vi "pmu_Write Physical Channel Info.vi"(8 "error in (no error)":errorcluster, 10 "physical channels":T1[](array[typedef]), 11 "system info in":refnum<class "PMU System Info.lvclass">) -> (0 "error out":errorcluster, 3 "system info out":refnum<class "PMU System Info.lvclass">)   [LabVIEW 2011, in "NI_EP_PMU.lvlib" / "PMU System Info.lvclass"]
uses:
  <vilib>/addons/Electrical Power/PMU/Common/Classes/PMU System Info/PMU System Info.lvclass
  <vilib>/addons/Electrical Power/PMU/Common/Controls/pmu_Physical Channel.ctl
  <vilib>/addons/Electrical Power/PMU/Common/Controls/pmu_Channel Phase.ctl
  <vilib>/addons/Electrical Power/PMU/Common/Classes/PMU System Info/PMU System Info.lvclass/PMU System Info.ctl
  <vilib>/addons/Electrical Power/PMU/NI_EP_PMU.lvlib
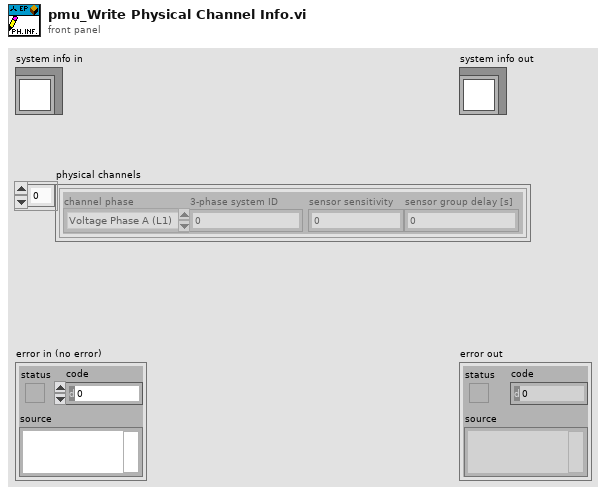
[diagram p1: front panel]
types:
  T1 = typedef "NI_EP_PMU.lvlib/pmu_Physical Channel.ctl" = cluster{"channel phase":T2, "3-phase system ID":u8, "sensor sensitivity":dbl, "sensor group delay [s]":dbl}
  T2 = typedef "NI_EP_PMU.lvlib/pmu_Channel Phase.ctl" = enum16{"Voltage Phase A (L1)", "Voltage Phase B (L2)", "Voltage Phase C (L3)", "Voltage Phase N (Neutral)", "Current Phase A (L1)", "Current Phase B (L2)", "Current Phase C (L3)", "Current Phase N (Neutral)"}
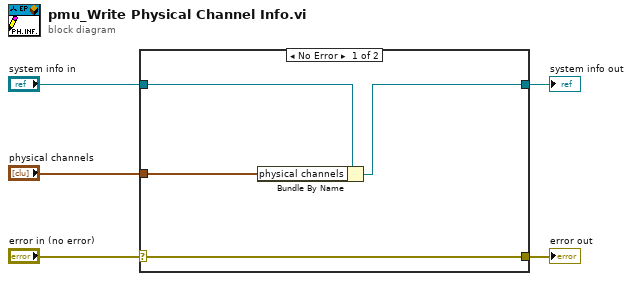
[diagram p0: block diagram]
diagram:
  n1 = case shown="No Error" "error in (no error)" {
    selector: "error in (no error)" -> [w9 w10]
    tunnel: [w9 w10] -> w4
    tunnel: [w6 w11] -> w2
    tunnel: "system info in" -> [w8 w11]
    tunnel: "physical channels" -> [w7 _]
    frame No Error {
      n2 = Bundle By Name(cluster=w8, "physical channels"=w7) -> (w6:refnum<class "PMU System Info.lvclass">)
    }
    frame Error {
    }
  }
  "error out" <- w4
  "system info out" <- w2
